vi "Target Vision Testing.vi"() -> ()   [LabVIEW 2013]
uses:
  <vilib>/Rock Robotics/WPI/Camera/WPI_CameraSettings Read MJPG.ctl
  <vilib>/Rock Robotics/WPI/Camera/WPI_CameraImageSize.ctl
  <vilib>/vision/Measure.llb/Edge Options.ctl
  <vilib>/vision/Measure.llb/Edge Polarity.ctl
  <vilib>/vision/Measure.llb/Straight Edge Options.ctl
  <vilib>/vision/Measure.llb/Straight Edge Process.ctl
  <vilib>/vision/NI_Vision_Development_Module.lvlib
panel:
  in  "Edge Options 2":T1={"Edge Polarity"=0, "Kernel Size"=3, "Width"=3, "Minimum Edge Strength"=10.0, "Interpolation Type"=enum."Bilinear Fixed", "Data Processing Method"=enum."Average"} {"Edge Polarity" items=["All Edges", "Rising Edges", "Falling Edges"]; "Minimum Edge Strength" format="%.2f"; "Width" step=2; "Kernel Size" step=2}
  in  "Line Options 2":T3={"Number of Lines"=1, "Type"=enum."Best Edge Projection", "Min. Score"=10.0, "Max. Score"=1000.0, "Orientation"=0.0, "Angle Range"=10.0, "Angle Tolerance"=1.0, "Step Size"=3, "Min. SNR (db)"=0.0, "Min. Points (%)"=25.0, "Hough Iterations"=5} {"Min. Points (%)" min=0.0 max=100.0; "Min. SNR (db)" min=0.0; "Max. Score" min=0.0 max=1024.0; "Min. Score" min=0.0 max=1024.0 step=1.0}
  in  "Line Options":T3={"Number of Lines"=1, "Type"=enum."Best Edge Projection", "Min. Score"=10.0, "Max. Score"=1000.0, "Orientation"=0.0, "Angle Range"=10.0, "Angle Tolerance"=1.0, "Step Size"=3, "Min. SNR (db)"=0.0, "Min. Points (%)"=25.0, "Hough Iterations"=5} {"Min. Points (%)" min=0.0 max=100.0; "Min. SNR (db)" min=0.0; "Max. Score" min=0.0 max=1024.0; "Min. Score" min=0.0 max=1024.0 step=1.0}
  in  "Edge Options":T1={"Edge Polarity"=0, "Kernel Size"=3, "Width"=3, "Minimum Edge Strength"=10.0, "Interpolation Type"=enum."Bilinear Fixed", "Data Processing Method"=enum."Average"} {"Edge Polarity" items=["All Edges", "Rising Edges", "Falling Edges"]; "Minimum Edge Strength" format="%.2f"; "Width" step=2; "Kernel Size" step=2}
  in  "Range":cluster{"Lower value":sgl, "Upper value":sgl}={"Lower value"=128.0, "Upper value"=255.0} {"Upper value" format="%.2f"; "Lower value" format="%.2f"}
  in  "stop":bool
  out "Image":T5(plugin-control)
  in  "Camera Settings":T6={"fps"=15, "compression"=5, "Image Size"=enum."320x240"}
  in  "Camera IP":string="10.00.00.11"
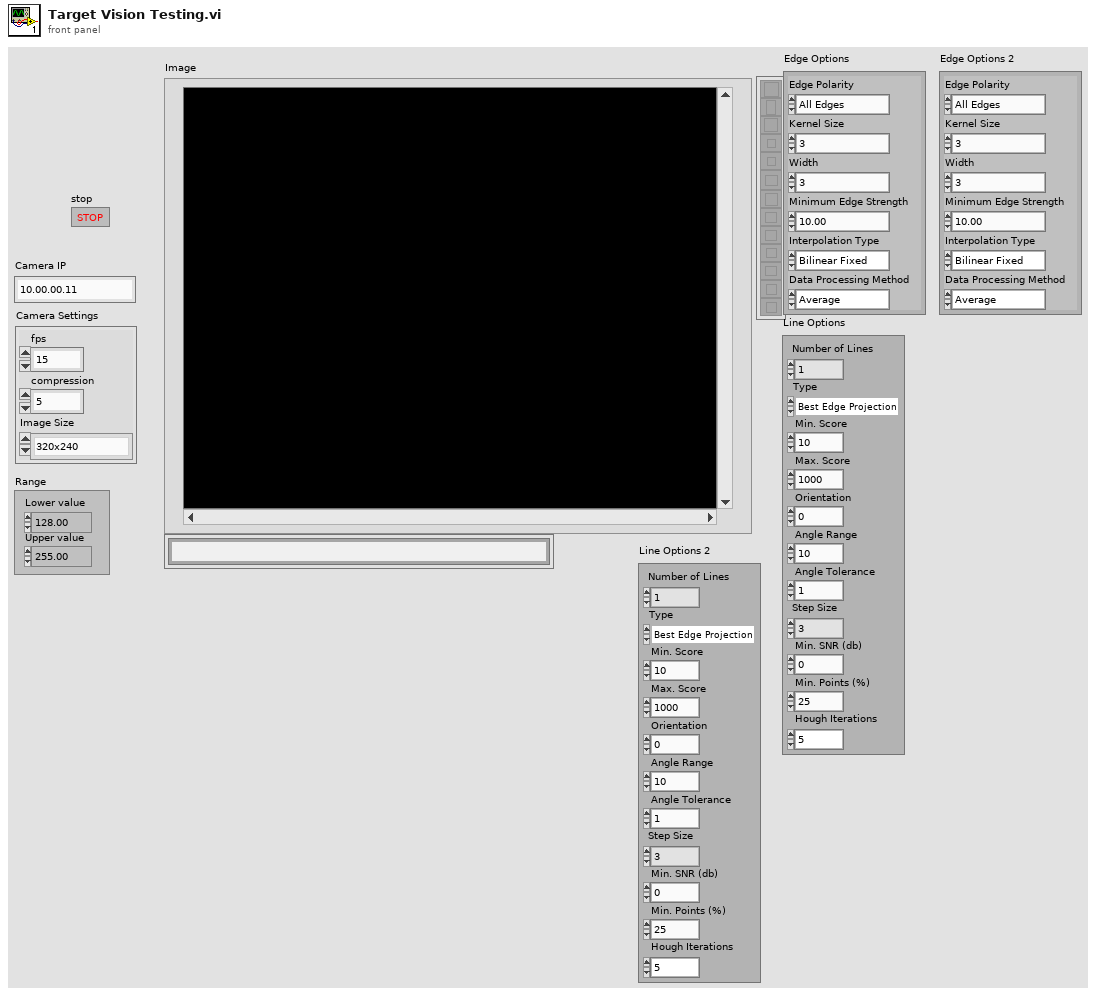
[diagram p1: front panel]
types:
  T1 = typedef "Edge Options.ctl" = cluster{"Edge Polarity":T2, "Kernel Size":u32, "Width":u32, "Minimum Edge Strength":sgl, "Interpolation Type":enum32{"Zero Order", "Bilinear", "Quadratic", "Cubic", "Bilinear Fixed"}, "Data Processing Method":enum32{"Average", "Median"}}
  T2 = typedef "Edge Polarity.ctl" = u32
  T3 = typedef "Straight Edge Options.ctl" = cluster{"Number of Lines":i32, "Type":T4, "Min. Score":dbl, "Max. Score":dbl, "Orientation":dbl, "Angle Range":dbl, "Angle Tolerance":dbl, "Step Size":u32, "Min. SNR (db)":dbl, "Min. Points (%)":dbl, "Hough Iterations":i32}
  T4 = typedef "Straight Edge Process.ctl" = enum32{"First Edge Rake", "Best Edge Rake", "Hough Edge Rake", "First Edge Projection", "Best Edge Projection"}
  T5 = typedef "IMAQ Image.ctl" = refnum<image>
  T6 = typedef "WPI_CameraSettings Read MJPG.ctl" = cluster{"fps":i32, "compression":i32, "Image Size":T7}
  T7 = typedef "WPI_CameraImageSize.ctl" = enum16{"640x480", "320x240", "160x120"}
  T8 = typedef "IMAQ Rectangle" = cluster{"Left":i32, "Top":i32, "Right":i32, "Bottom":i32, "Rotation":dbl}
  T9 = typedef "Image Type" = u32
  T10 = typedef "ROI Descriptor" = cluster{"Global Rectangle":i32[], "Contours":cluster{"ID":enum32{"External", "Internal"}, "Type":u32, "Coordinates":i32[]}[]}
  T11 = cluster{"Global Rectangle":i32[], "Contours":cluster{"Contour Type":u32, "ROI Type":u32, "Points":i32[]}[]}
  T12 = cluster{"Point1 (Pixels)":cluster{"X":sgl, "Y":sgl}, "Point2 (Pixels)":cluster{"X":sgl, "Y":sgl}, "Point1 (Real-World)":cluster{"X":sgl, "Y":sgl}, "Point2 (Real-World)":cluster{"X":sgl, "Y":sgl}, "Angle (Pixel)":dbl, "Angle (Real-World)":dbl, "Score":dbl, "Straightness":dbl, "Average SNR (db)":dbl, "Calibration Valid":bool}[]
  T13 = cluster{"Point1 (Pixels)":cluster{"X":sgl, "Y":sgl}, "Point2 (Pixels)":cluster{"X":sgl, "Y":sgl}, "Point1 (Real-World)":cluster{"X":sgl, "Y":sgl}, "Point2 (Real-World)":cluster{"X":sgl, "Y":sgl}, "Angle (Pixel)":dbl, "Angle (Real-World)":dbl, "Score":dbl, "Straightness":dbl, "Average SNR (db)":dbl, "Calibration Valid":bool}
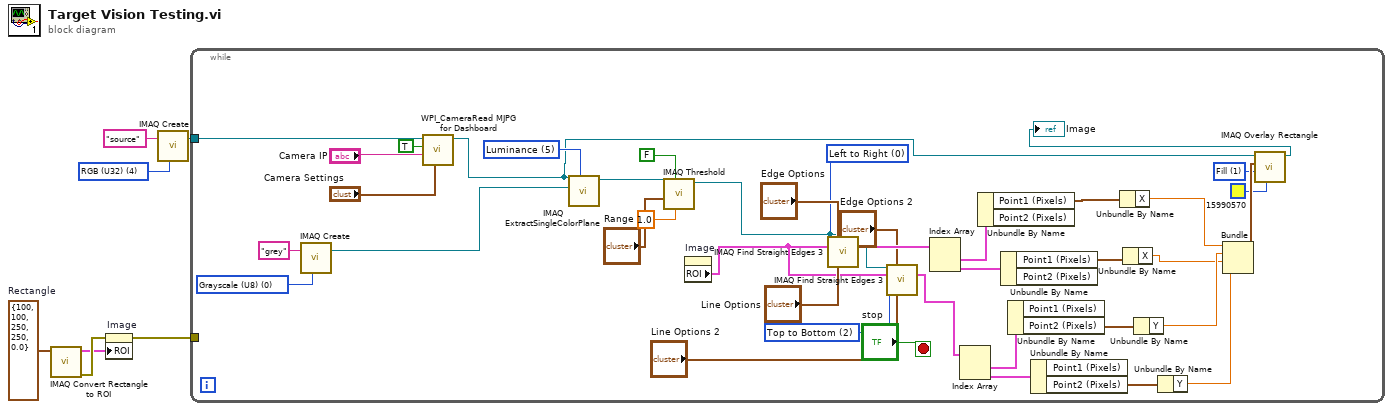
[diagram p0: block diagram]
diagram:
  w4 = T8 {"Left"=100, "Top"=100, "Right"=250, "Bottom"=250, "Rotation"=0.0}  # Rectangle
  w5 = T9 4 items=["Grayscale (U8)", "Grayscale (I16)", "Grayscale (SGL)", "Complex (CSG)", "RGB (U32)", "HSL (U32)", "RGB (U64)", "Grayscale (U16)"] ("Image Type")
  n1 = call "IMAQ Convert Rectangle to ROI"("Rectangle"=w4) -> ("error out"=w3:errorcluster, "ROI Descriptor"=w2:T10)  [unwired: 8 in]
  n2 = property on="Image" class="ImageControl"(error in=w3, "ROI"=w2) -> (error out=w1:errorcluster)  [unwired: 1 in, 1 out]
  n3 = call "IMAQ Create"("Image Name"="source", "Image Type"=w5) -> ("New Image"=w6:T5)  [unwired: 3 in, 1 out]
  n4 = while {
    tunnel: w6 -> [w43]
    tunnel: w1 -> [_]
    stop <- "stop" stop-if-true
    w8 = u32 1 items=["Frame", "Fill", "Highlight"] ("Drawing Mode (Frame)")
    w32 = u32 0 items=["Left to Right", "Right to Left", "Top to Bottom", "Bottom to Top"] ("Search Direction")
    w29 = u32 2 items=["Left to Right", "Right to Left", "Top to Bottom", "Bottom to Top"] ("Search Direction")
    w41 = T9 0 items=["Grayscale (U8)", "Grayscale (I16)", "Grayscale (SGL)", "Complex (CSG)", "RGB (U32)", "HSL (U32)", "RGB (U64)", "Grayscale (U16)"] ("Image Type")
    w42 = 5 items=["Red", "Green", "Blue", "Hue", "Saturation", "Luminance", "Value", "Intensity"] ("Color Plane")
    n5 = call "IMAQ Create"("Image Name"="grey", "Image Type"=w41) -> ("New Image"=w39:T5)  [unwired: 3 in, 1 out]
    n6 = call <vilib>:"WPI_CameraRead MJPG for Dashboard.vi"("Camera Settings"="Camera Settings", "Camera IP"="Camera IP", "Enable"=TRUE, "Refnum in"=w43) -> ("Refnum out"=w17:T5)  [unwired: 4 in, 3 out]
    n7 = call "IMAQ ExtractSingleColorPlane"("Color Plane"=w42, "Image Dst"=w39, "Image Src"=w17) -> ("Image Dst Out"=w38:T5)  [unwired: 7 in, 1 out]
    n8 = call "IMAQ Threshold"("Replace Value"=sgl 1.0, "Keep/Replace Value (Replace)"=FALSE, "Range"="Range", "Image Src"=w38) -> ("Image Dst Out"=w31:T5)  [unwired: 6 in, 1 out]
    n9 = property on="Image" class="ImageControl"() -> ("ROI"=w30:T11)  [unwired: 2 in, 2 out]
    n10 = call "IMAQ Find Straight Edges 3"("Image"=w31, "Edge Options"="Edge Options", "ROI Descriptor"=w30, "Search Direction"=w32, "Line Options"="Line Options") -> ("Straight Edges"=w27:T12)  [unwired: 6 in, 4 out]
    n11 = call "IMAQ Find Straight Edges 3"("Image"=w31, "Edge Options"="Edge Options 2", "ROI Descriptor"=w30, "Search Direction"=w29, "Line Options"="Line Options 2") -> ("Straight Edges"=w22:T12)  [unwired: 6 in, 4 out]
    n12 = Index Array(array=w27) -> (element #1=w26:T13, element #2=w25:T13)  [unwired: 2 in]
    n13 = Index Array(array=w22) -> (element #1=w24:T13, element #2=w23:T13)  [unwired: 2 in]
    n14 = Unbundle By Name(w26) -> ("Point1 (Pixels)"=w21:cluster{"X":sgl, "Y":sgl})  [unwired: 1 out]
    n15 = Unbundle By Name(w25) -> ("Point1 (Pixels)"=w20:cluster{"X":sgl, "Y":sgl})  [unwired: 1 out]
    n16 = Unbundle By Name(w24) -> ("Point2 (Pixels)"=w18:cluster{"X":sgl, "Y":sgl})  [unwired: 1 out]
    n17 = Unbundle By Name(w23) -> ("Point2 (Pixels)"=w19:cluster{"X":sgl, "Y":sgl})  [unwired: 1 out]
    n18 = Unbundle By Name(w21) -> ("X"=w16:sgl)
    n19 = Unbundle By Name(w20) -> ("X"=w14:sgl)
    n20 = Unbundle By Name(w18) -> ("Y"=w15:sgl)
    n21 = Unbundle By Name(w19) -> ("Y"=w13:sgl)
    n22 = Bundle("X"=w16, "Y"=w15, "X"=w14, "Y"=w13) -> (w12:cluster{"X":sgl, "Y":sgl, "X":sgl, "Y":sgl})  [unwired: 1 in]
    n23 = call "IMAQ Overlay Rectangle"("Color"=u32 15990570, "Drawing Mode (Frame)"=w8, "Rectangle"=w12, "Image"=w17) -> ("Image Out"=→"Image":T5)  [unwired: 6 in, 1 out]
  }
